vi "Read UUT Data.vi"(8 "error in (no error)":errorcluster, 10 "Number Bytes To Read (256)":i32=256, 11 "VISA resource name":refnum<visa-resource-name>) -> (0 "error out":errorcluster, 1 "UUT Data":string, 2 "NumBytes Read":i32, 3 "VISA resource name out":refnum<visa-resource-name>)   [LabVIEW 2014, in "Fluke 5XXX Series Multicalibrators.lvlib"]
doc: "This VI returns data from the UUT in IEEE-488.2 Standard format over the Calibrator rear panel SERIAL 2 TO UUT serial port. The command may be sent over gpib or RS-232 ports, but applies to SERIAL 2 TO UUT serial port operation.\n\nNote:\n\nThis VI is available only for instrument models 5500A and 5520A."
uses:
  Fluke 5XXX Series Multicalibrators.lvlib
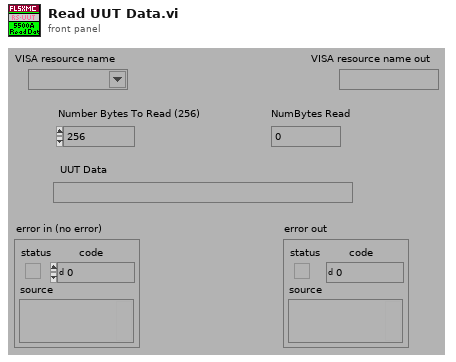
[diagram p1: front panel]
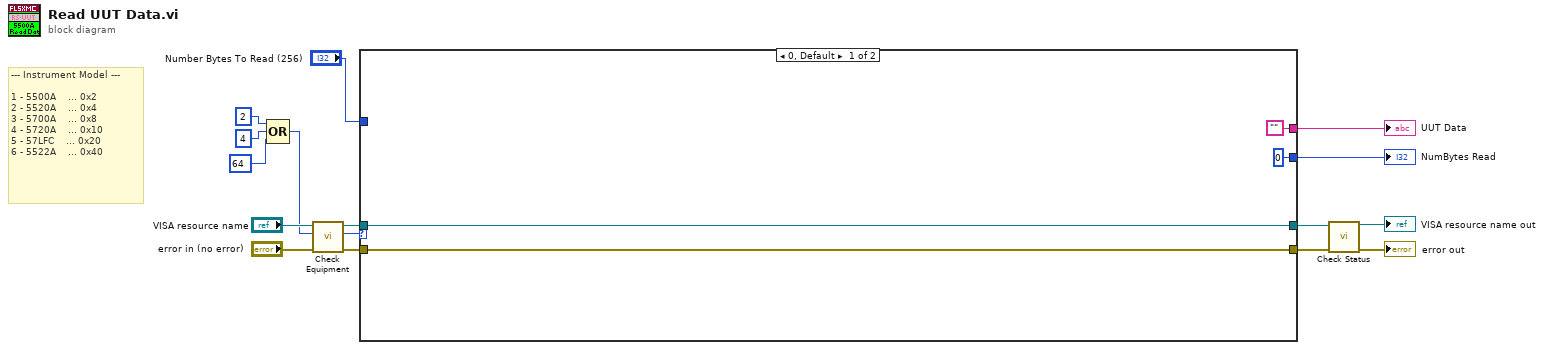
[diagram p0: block diagram]
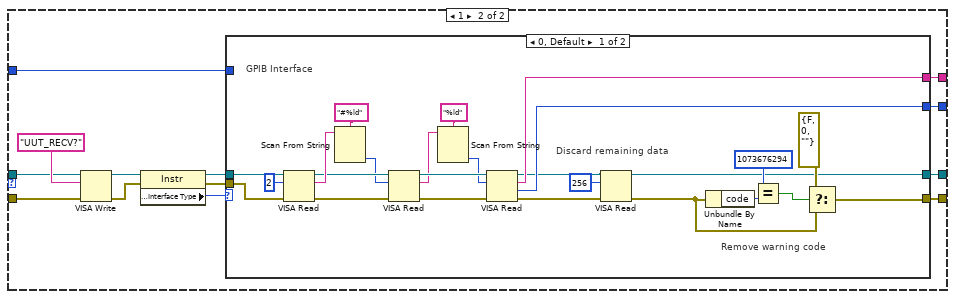
[diagram p2: hidden frame]
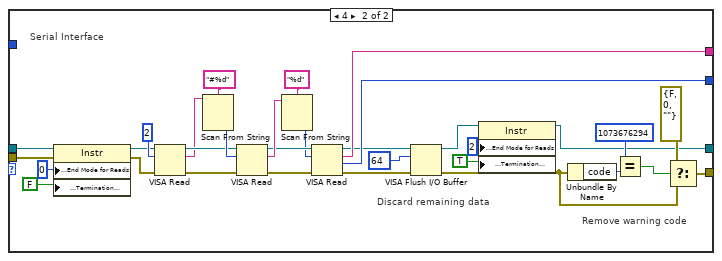
[diagram p3: hidden frame]
diagram:
  # "--- Instrument Model ---\n\n1 - 5500A    ... 0x2\n2 - 5520A    ... 0x4\n3 - 5700A    ... 0x8\n4 - 5720A    ... 0x10\n5 - 57LFC    ... 0x20\n6 - 5522A    ... 0x40"
  n1 = Compound Arithmetic op=OR(u32 2, u32 4, 64 ("Numeric")) -> (w12:u32)
  n2 = call "Check Equipment.vi"("error in (no error)"="error in (no error)", "Bit Mask"=w12, "VISA resource name"="VISA resource name") -> ("error out"=w16:errorcluster, "Present?"=w9:u32, "VISA resource name out"=w15:refnum<visa-resource-name>)  [unwired: 6 in]
  n3 = case shown="0, Default" w9 {
    tunnel: w16 -> [w19 w30]
    tunnel: w15 -> [w20 w29]
    tunnel: [w20 w24] -> w5
    tunnel: [w19 w23] -> w3
    tunnel: "Number Bytes To Read (256)" -> [_ w25]
    tunnel: ["" w22] -> w7
    tunnel: [u32 0 ("return count") w21] -> w6
    frame 0, Default {
    }
    frame 1 {
      n4 = VISA Write(VISA resource name=w29, write buffer="UUT_RECV?" ("write buffer (\"\")"), error in (no error)=w30) -> (VISA resource name out=w32:refnum<visa-resource-name>, error out=w31:errorcluster)  [unwired: 1 out]
      n5 = property class="Instr"(reference=w32, error in=w31) -> (reference out=w27:refnum<visa-resource-name>, error out=w26:errorcluster, "Interface Information:Interface Type"=w28:u16)
      n6 = case shown="0, Default" w28 {
        tunnel: w27 -> [w58 w70]
        tunnel: w26 -> [w57 w69]
        tunnel: w25 -> [_ _]
        tunnel: [w36 w68] -> w24
        tunnel: [w41 w67] -> w23
        tunnel: [w53 w65] -> w22
        tunnel: [w39 w66] -> w21
        frame 0, Default {
          # "Discard remaining data"
          # "Remove warning code"
          # "GPIB Interface"
          n7 = VISA Read(VISA resource name=w58, byte count=u32 2 ("byte count (0)"), error in (no error)=w57) -> (VISA resource name out=w50:refnum<visa-resource-name>, read buffer=w54:string, error out=w52:errorcluster)  [unwired: 1 out]
          n8 = Scan From String(format string="#%ld", input string=w54) -> (output 1=w46:i32)  [unwired: 3 in, 3 out]
          n9 = VISA Read(VISA resource name=w50, byte count=w46, error in (no error)=w52) -> (VISA resource name out=w48:refnum<visa-resource-name>, read buffer=w47:string, error out=w51:errorcluster)  [unwired: 1 out]
          n10 = Scan From String(format string="%ld", input string=w47) -> (output 1=w40:i32)  [unwired: 3 in, 3 out]
          n11 = VISA Read(VISA resource name=w48, byte count=w40, error in (no error)=w51) -> (VISA resource name out=w37:refnum<visa-resource-name>, read buffer=w53:string, return count=w39:u32, error out=w38:errorcluster)
          n12 = VISA Read(VISA resource name=w37, byte count=u32 256 ("byte count (0)"), error in (no error)=w38) -> (VISA resource name out=w36:refnum<visa-resource-name>, error out=w35:errorcluster)  [unwired: 2 out]
          n13 = Unbundle By Name(w35) -> ("code"=w42:i32)
          n14 = Equal?(x=1073676294, y=w42) -> (x = y?=w44:bool)
          n15 = Select(t=errorcluster {"status"=FALSE, "code"=0, "source"=""} ("error out"), s=w44, f=w35) -> (s? t:f=w41:errorcluster)
        }
        frame 4 {
          # "Discard remaining data"
          # "Remove warning code"
          # "Serial Interface"
          n16 = property class="Instr"(reference=w70, error in=w69, "Serial Settings:End Mode for Reads"=u16 0 ("ASRL End In"), "Message Based Settings:Termination Character Enable"=FALSE ("TermChar En")) -> (reference out=w77:refnum<visa-resource-name>, error out=w78:errorcluster)
          n17 = VISA Read(VISA resource name=w77, byte count=u32 2 ("byte count (0)"), error in (no error)=w78) -> (VISA resource name out=w82:refnum<visa-resource-name>, read buffer=w81:string, error out=w83:errorcluster)  [unwired: 1 out]
          n18 = Scan From String(format string="#%d", input string=w81) -> (output 1=w84:i32)  [unwired: 3 in, 3 out]
          n19 = VISA Read(VISA resource name=w82, byte count=w84, error in (no error)=w83) -> (VISA resource name out=w73:refnum<visa-resource-name>, read buffer=w85:string, error out=w74:errorcluster)  [unwired: 1 out]
          n20 = Scan From String(format string="%d", input string=w85) -> (output 1=w64:i32)  [unwired: 3 in, 3 out]
          n21 = VISA Read(VISA resource name=w73, byte count=w64, error in (no error)=w74) -> (VISA resource name out=w63:refnum<visa-resource-name>, read buffer=w65:string, return count=w66:u32, error out=w62:errorcluster)
          n22 = VISA Flush I/O Buffer(VISA resource name=w63, mask (16)=u32 64, error in (no error)=w62) -> (VISA resource name out=w60:refnum<visa-resource-name>, error out=w61:errorcluster)
          n23 = property class="Instr"(reference=w60, "Serial Settings:End Mode for Reads"=u16 2 ("ASRL End In"), "Message Based Settings:Termination Character Enable"=TRUE ("TermChar En")) -> (reference out=w68:refnum<visa-resource-name>)  [unwired: 1 in, 1 out]
          n24 = Unbundle By Name(w61) -> ("code"=w87:i32)
          n25 = Equal?(x=1073676294, y=w87) -> (x = y?=w89:bool)
          n26 = Select(t=errorcluster {"status"=FALSE, "code"=0, "source"=""} ("error out"), s=w89, f=w61) -> (s? t:f=w67:errorcluster)
        }
      }
    }
  }
  "UUT Data" <- w7
  "NumBytes Read" <- w6
  n27 = call "Check Status.vi"("VISA resource name"=w5, "error in (no error)"=w3) -> ("VISA resource name out"=→"VISA resource name out":refnum<visa-resource-name>, "error out"=→"error out":errorcluster)  [unwired: 12 in]
